vi "Solution part 1a.vi"(11 "data?":bool) -> ()   [LabVIEW 2020]
panel:
  out "mask":u64 format="%.0x"
  out "sum of memory":u64
  out "mask for resetting":u64 format="%.0b"
  out "mask for setting":u64 format="%.0b"
  out "mask len ok?":bool
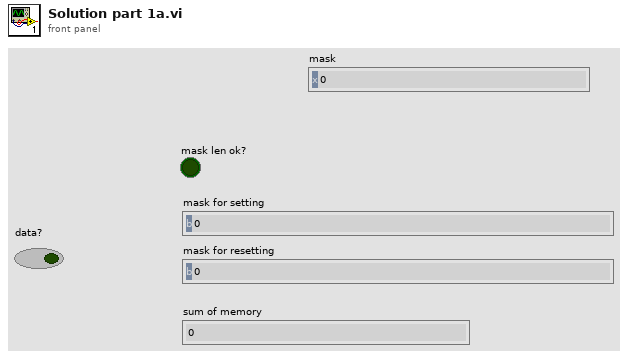
[diagram p1: front panel]
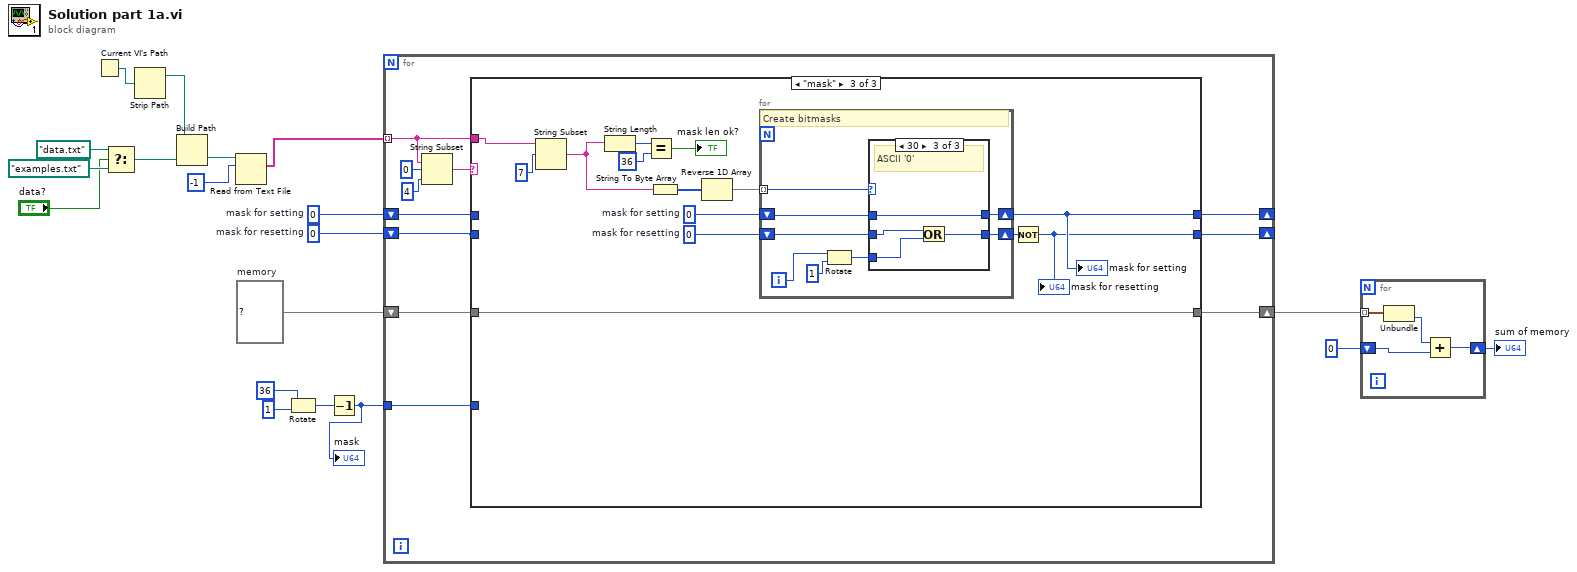
[diagram p0: block diagram]
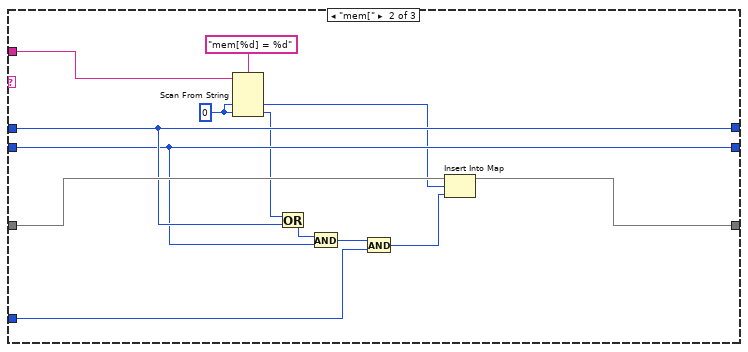
[diagram p3: hidden frame]
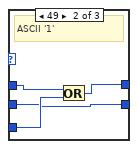
[diagram p5: hidden frame]
diagram:
  w8 = u64 0  # mask for setting
  w7 = u64 0  # mask for resetting
  w6 = map{u64, u64} {}  # memory
  n1 = Current VI's Path() -> (path=w16:path)
  n2 = Select(t=path "data.txt", s="data?", f=path "examples.txt") -> (s? t:f=w17:path)
  n3 = Strip Path(path=w16) -> (stripped path=w15:path)  [unwired: 1 out]
  n4 = Build Path(base path=w15, name or relative path=w17) -> (appended path=w14:path)
  n5 = Read from Text File(file (use dialog)=w14, count=-1) -> (text=w9:string[])  [unwired: 2 in, 3 out]
  n6 = Rotate(1:u64 1 ("x"), 2:i16 36 ("y")) -> (0:w2:u64)
  n7 = Decrement(x=w2) -> (x-1=w1:u64)
  "mask" <- w1
  n8 = for {
    tunnel: w9 -> [w21] mode=indexing
    shift-right: [w24] -> _
    shift-left: w7 -> [w26]
    shift-right: [w25] -> _
    shift-left: w8 -> [w27]
    shift-right: [w22] -> w5
    shift-left: w6 -> [w23]
    tunnel: w1 -> [w20]
    n9 = String Subset(string=w21, offset (0)=0, length (rest)=4 ("length (rest)")) -> (substring=w28:string)
    n10 = case shown="\"mask\"" w28 {
      tunnel: w27 -> [w33 w45 _]
      tunnel: w26 -> [w32 w44 _]
      tunnel: [w33 w45 w53] -> w25
      tunnel: [w32 w44 w51] -> w24
      tunnel: w23 -> [w31 w46 w50]
      tunnel: [w31 w43 w50] -> w22
      tunnel: w21 -> [_ w36 w49]
      tunnel: w20 -> [_ w34 _]
      frame Default {
      }
      frame "mem[" {
        w40 = u64 0 ("default value 2")
        n11 = Scan From String(format string="mem[%d] = %d", input string=w36, default 1=w40, default 2=w40) -> (output 1=w38:u64, output 2=w41:u64)  [unwired: 2 in, 3 out]
        n12 = Or(x=w41, y=w45) -> (x .or. y?=w39:u64)
        n13 = And(x=w39, y=w44) -> (x .and. y?=w37:u64)
        n14 = And(x=w37, y=w34) -> (x .and. y?=w35:u64)
        n15 = Insert Into Map(map in=w46, key=w38, value=w35) -> (map out=w43:map{u64, u64})  [unwired: 2 out]
      }
      frame "mask" {
        w48 = u64 0  # mask for setting
        w47 = u64 0  # mask for resetting
        n16 = String Subset(string=w49, offset (0)=7) -> (substring=w57:string)  [unwired: 1 in]
        n17 = String Length(string=w57) -> (length=w58:i32)
        n18 = Equal?(x=w58, y=36) -> (x = y?=→"mask len ok?":bool)
        n19 = String To Byte Array(string=w57) -> (unsigned byte array=w56:u8[])
        n20 = Reverse 1D Array(array=w56) -> (reversed array=w60:u8[])
        n21 = for {
          tunnel: w60 -> [w68] mode=indexing
          shift-right: [w63] -> w53
          shift-left: w48 -> [w67]
          shift-right: [w61] -> w52
          shift-left: w47 -> [w62]
          i -> [w65]
          # "Create bitmasks"
          n22 = Rotate(1:u64 1 ("x"), 2:w65) -> (0:w64:u64)
          n23 = case shown="30" w68 {
            tunnel: w67 -> [w70 w74 w75]
            tunnel: w64 -> [_ w73 w78]
            tunnel: [w70 w72 w75] -> w63
            tunnel: w62 -> [w69 w71 w77]
            tunnel: [w69 w71 w76] -> w61
            frame Default {
              # "Ignore the rest"
            }
            frame 49 {
              # "ASCII '1'"
              n24 = Or(x=w74, y=w73) -> (x .or. y?=w72:u64)
            }
            frame 48 {
              # "ASCII '0'"
              n25 = Or(x=w77, y=w78) -> (x .or. y?=w76:u64)
            }
          }
        }
        "mask for setting" <- w53
        n26 = Not(x=w52) -> (.not. x?=w51:u64)
        "mask for resetting" <- w51
      }
    }
  }
  n27 = for {
    shift-right: [w82] -> w10
    shift-left: u64 0 ("default value 2") -> [w80]
    tunnel: w5 -> [w79] mode=indexing
    n28 = Unbundle(w79) -> (w81:u64)  [unwired: 1 out]
    n29 = Add(x=w81, y=w80) -> (x+y=w82:u64)
  }
  "sum of memory" <- w10
